vi "Set Type Varies.vi"(7 "caller name":string, 8 "error in (no error)":errorcluster) -> (0 "error out":errorcluster)   [LabVIEW 2016, in "CVT.lvlib" / "Current Value Table.lvlib"]
doc: "This is simply a holder for error 537166 and does not have any other functionality."
uses:
  Current Value Table.lvlib
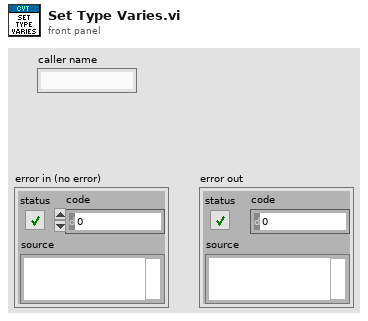
[diagram p1: front panel]
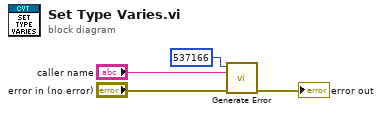
[diagram p0: block diagram]
diagram:
  n1 = call "Generate Error.vi"("error in"="error in (no error)", "caller name"="caller name", "code"=537166) -> ("error out"=→"error out":errorcluster)  [unwired: 8 in]
